vi "Empty String Replacement.vi"(7 "Empty":string, 11 "String":string) -> (3 "String Out":string)   [LabVIEW 2023, in "VIDoc Printer.lvlib" / "VIDoc Printer.lvclass"]
doc: "If String is empty, it instead outputs the value under Empty."
uses:
  VIDoc Printer.lvclass
  VIDoc Printer.lvclass/VIDoc Printer.ctl
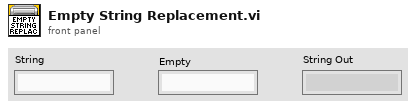
[diagram p1: front panel]
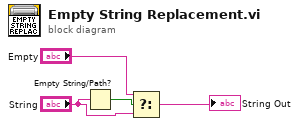
[diagram p0: block diagram]
diagram:
  n1 = Empty String/Path?(string/path="String") -> (empty?=w3:bool)
  n2 = Select(t="Empty", s=w3, f="String") -> (s? t:f=→"String Out":string)
